vi "poster1.vi"(4 "error in":errorcluster, 7 "file path":path) -> (0 "error out":errorcluster, 1 "last ses time":timestamp caption="отправлено на SMGR", 2 "Tab Control":enum32{"ГП", "КР"}(tab), 3 "file dup":path)   [LabVIEW 2010]
uses:
  Global 2.vi
  <vilib>/measure/matone.llb/Extract Single Tone Information 1 Chan.vi
  <vilib>/measure/NI_MAPro.lvlib
panel:
  out "phase (deg)":dbl format="%.2p"
  out "frequency":dbl format="%.2p"
  in  "s":bool=TRUE caption="нач\\всё"
  out "wgp1":waveform(i16)[](graph) caption="C:\\Users\\USER\\AppData\\Local\\Temp\\12-2011_07_12-06_42_24_7.dat"
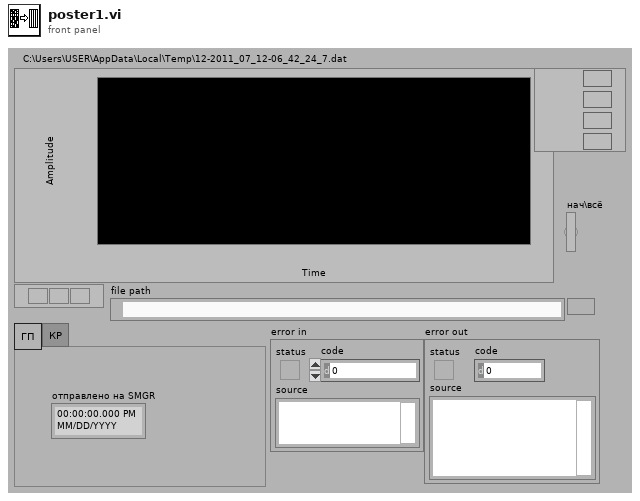
[diagram p1: front panel]
types:
  T1 = cluster{"DeviceID":i32, "DeviceDateTimeUTC":timestamp, "log":string[], "SMGR2 FilePath":path, "table FilePath":path}
  T2 = cluster{"App:Default Data Directory":path, "seconds since 1Jan1904":timestamp, "name or relative path":string}
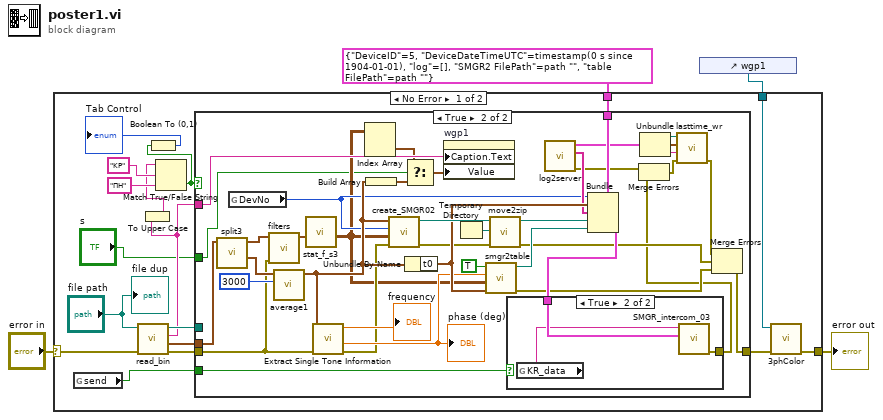
[diagram p0: block diagram]
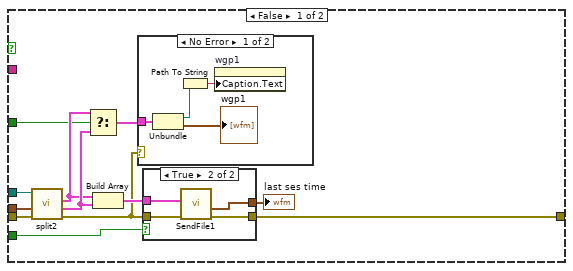
[diagram p2: hidden frame]
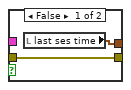
[diagram p3: hidden frame]
diagram:
  n1 = control-ref of="wgp1"() -> (w1:refnum<vi>)
  n2 = case shown="No Error" "error in" {
    selector: "error in" -> [w14 w86]
    tunnel: [w6 w86] -> w4
    tunnel: T1 {"DeviceID"=5, "DeviceDateTimeUTC"=timestamp(0 s since 1904-01-01), "log"=[], "SMGR2 FilePath"=path "", "table FilePath"=path ""} ("InputData") -> [w9 _]
    tunnel: w1 -> [w8 _]
    frame No Error {
      n3 = global read "Global 2.vi" "send"() -> (w13:bool)
      n4 = call "read_bin.vi"("error in"=w14, "datalog path"="file path") -> ("error out"=w20:errorcluster, "Waveform Graph"=w21:waveform(i16)[], "group name"=w15:string, "new file path"=w19:path)  [unwired: 2 in]
      n5 = To Upper Case(1:w15) -> (0:w16:string)
      n6 = Match True/False String(2:"ПН" ("true string"), 3:"KP" ("true string"), 4:w16) -> (0:w11:bool)  [unwired: 1 out]
      n7 = Boolean To (0,1)(Boolean=w11) -> (0, 1=→"Tab Control":i16)
      n8 = case shown="True" w11 {
        tunnel: [w33 w46] -> w7
        tunnel: w21 -> [w32 w82]
        tunnel: w20 -> [w31 w44]
        tunnel: w19 -> [w30 _]
        tunnel: w15 -> [_ w71]
        tunnel: w13 -> [w23 w62]
        tunnel: w9 -> [_ w76]
        tunnel: "s" -> [w22 w47]
        frame False {
          n9 = call "split2.vi"("error in"=w31, "Waveforms"=w32, "full file path"=w30) -> ("error out"=w25:errorcluster, "compressed"=w28:cluster{"appended path":path, waveform(i16)[]}, "first"=w27:cluster{"appended path":path, waveform(i16)[]})  [unwired: 2 in]
          n10 = Select(t=w27, s=w22, f=w28) -> (s? t:f=w26:cluster{"appended path":path, waveform(i16)[]})
          n11 = Build Array(w27, w28) -> (w29:cluster{"appended path":path, waveform(i16)[]}[])
          n12 = case shown="No Error" w25 {
            tunnel: w26 -> [w43 _]
            frame No Error {
              n13 = Unbundle(w43) -> ("appended path"=w41:path, →"wgp1":waveform(i16)[])
              n14 = Path To String(path=w41) -> (string=w40:string)
              n15 = property on="wgp1" class="WFGraph (strict)"("Caption.Text"=w40) -> ()  [unwired: 2 in, 2 out]
            }
            frame Error {
            }
          }
          n16 = case shown="True" w23 {
            tunnel: [w35 w39] -> w33
            tunnel: w29 -> [_ w38]
            tunnel: w25 -> [w35 w37]
            tunnel: [w34 w36] -> w24
            frame False {
              n17 = local read "last ses time"() -> (w34:timestamp)
            }
            frame True {
              n18 = call "SendFile1.vi"("error in"=w37, "Array"=w38) -> ("error out"=w39:errorcluster, "last ses time"=w36:timestamp)  [unwired: 4 in]
            }
          }
          "last ses time" <- w24
        }
        frame True {
          n19 = call "split3.vi"("Array of Waveform In"=w82) -> ("Sync"=w81:waveform(i16), "Array of Waveform"=w79:waveform(i16)[])  [unwired: 5 in]
          n20 = global read "Global 2.vi" "DevNo"() -> (w52:i32)
          n21 = call "filters.vi"("error in (no error)"=w44, "Array"=w79) -> ("Array 2"=w78:waveform(i16)[])  [unwired: 5 in]
          n22 = call "average1.vi"("Size"=3000, "SignalIn"=w81) -> ("output waveform"=w70:waveform(i16))  [unwired: 5 in]
          n23 = call "stat_f_s3.vi"("Array of Wfm"=w78) -> ("Array 2"=w51:waveform(i16)[][])  [unwired: 6 in]
          n24 = call-poly <vilib>:"Extract Single Tone Information.vi"("error in (no error)"=w44, "time signal in"=w70) -> ("error out"=w61:errorcluster, "detected phase (deg)"=w68:dbl, "detected frequency"=→"frequency":dbl)  [unwired: 4 in, 3 out]
          "phase (deg)" <- w68
          n25 = Index Array(array=w51) -> (element=w50:waveform(i16)[])  [unwired: 2 in]
          n26 = Build Array(w70) -> (w49:waveform(i16)[])
          n27 = call "create_SMGR02.vi"("error out in"=w61, "array"=w51, "meas_point"=w52, "sync"=w70) -> ("error out"=w64:errorcluster, "path"=w75:path)  [unwired: 4 in]
          n28 = Select(t=w50, s=w47, f=w49) -> (s? t:f=w48:waveform(i16)[])
          n29 = Unbundle By Name(w70) -> ("t0"=w69:timestamp)
          n30 = property on="wgp1" class="WFGraph (strict)"("Caption.Text"=w71, "Value"=w48) -> ()  [unwired: 2 in, 2 out]
          n31 = Temporary Directory() -> (w73:path)
          n32 = call "smgr2table.vi"("t0"=w69, "Array 2"=w51, "detected phase (deg)"=w68, "write2file"=TRUE) -> ("error out"=w65:errorcluster, "zipped path"=w67:path)  [unwired: 2 out]
          n33 = call "move2zip.vi"("error in"=w64, "dest dir"=w73, "source path"=w75) -> ("error out"=w63:errorcluster, "zipped path"=w74:path)  [unwired: 3 in]
          n34 = call "log2server.vi"() -> ("error out"=w58:errorcluster, "msgs"=w60:string[], "cluster"=w56:T2)  [unwired: 5 in]
          n35 = Bundle(cluster=w76, "DeviceID"=w52, "DeviceDateTimeUTC"=w69, "log"=w60, "SMGR2 FilePath"=w74, "table FilePath"=w67) -> (w72:T1)
          n36 = case shown="True" w62 {
            tunnel: [_ w85] -> w59
            tunnel: w72 -> [_ w84]
            frame False {
            }
            frame True {
              n37 = global read "Global 2.vi" "KR_data"() -> (w83:string)
              n38 = call "SMGR_intercom_03.vi"("InputData"=w84, "URL:port"=w83) -> ("error out"=w85:errorcluster)  [unwired: 9 in]
            }
          }
          n39 = Merge Errors(w58, w59) -> (w57:errorcluster)
          n40 = Unbundle(w56) -> ("App:Default Data Directory"=w55:path, "seconds since 1Jan1904"=w54:timestamp, "name or relative path"=w53:string)
          n41 = call "lasttime_wr.vi"("error in"=w57, "name"=w53, "time stamp"=w54, "start Path"=w55) -> ("error out"=w45:errorcluster)  [unwired: 2 in, 1 out]
          n42 = Merge Errors(w45, w63, w65) -> (w46:errorcluster)
        }
      }
      n43 = call "3phColor.vi"("error in (no error)"=w7, "Waveform Graph"=w8) -> ("error out"=w6:errorcluster)  [unwired: 5 in]
      "file dup" <- "file path"
    }
    frame Error {
    }
  }
  "error out" <- w4
